vi "Get Screen BD Object Bounds.vi"(9 "Object Reference":refnum<vi>, 10 "BD Window Bounds":T1, 11 "BD Origin":T2) -> (1 "Object Visible?":bool, 2 "Screen Object Bounds":T1, 3 "Screen BD Bounds":T1)   [LabVIEW 2019, in "Window.lvlib"]
doc: "Converts the given block diagram coordinates into screen coordinates. Also converts the given object's size and position from block diagram coordinates to screen coordinates. The object is also checked for visibility on the block diagram window."
uses:
  <vilib>/Utility/miscctls.llb/LVPointTypeDef.ctl
  <vilib>/Utility/miscctls.llb/LVRectTypeDef.ctl
  Window.lvlib
  _2D/2D.lvlib
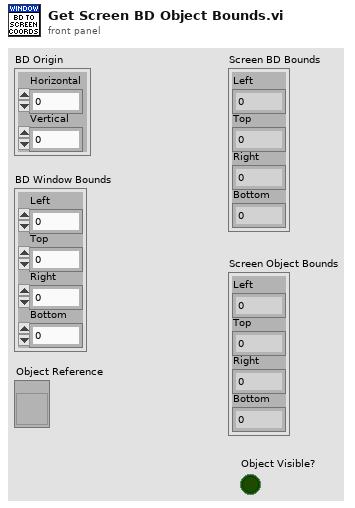
[diagram p1: front panel]
types:
  T1 = typedef "LVRectTypeDef.ctl" = cluster{"Left":i16, "Top":i16, "Right":i16, "Bottom":i16}
  T2 = typedef "LVPointTypeDef.ctl" = cluster{"Horizontal":i16, "Vertical":i16}
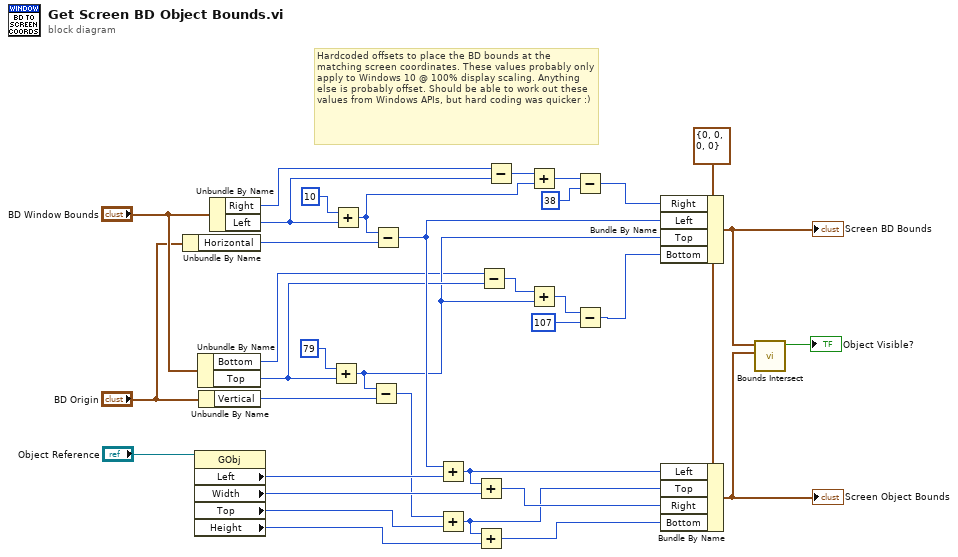
[diagram p0: block diagram]
diagram:
  w26 = T1 {"Left"=0, "Top"=0, "Right"=0, "Bottom"=0} ("Screen BD Bounds")
  # "Hardcoded offsets to place the BD bounds at the matching screen coordinates. These values probably only apply to Windows 10 @ 100% display scaling. Anything else is probably offset. Should be able to work out these values from Windows APIs, but hard coding was quicker :)"
  n1 = Unbundle By Name("BD Origin") -> ("Horizontal"=w29:i16)
  n2 = property class="GObj"(reference="Object Reference") -> ("Left"=w33:i32, "Width"=w32:u32, "Top"=w31:i32, "Height"=w30:u32)  [unwired: 1 in, 2 out]
  n3 = Unbundle By Name("BD Window Bounds") -> ("Bottom"=w5:i16, "Top"=w15:i16)
  n4 = Unbundle By Name("BD Origin") -> ("Vertical"=w27:i16)
  n5 = Unbundle By Name("BD Window Bounds") -> ("Right"=w6:i16, "Left"=w19:i16)
  n6 = Add(x=i16 79 ("y"), y=w15) -> (x+y=w13:i16)
  n7 = Add(x=i16 10, y=w19) -> (x+y=w7:i16)
  n8 = Subtract(x=w13, y=w27) -> (x-y=w20:i16)
  n9 = Subtract(x=w7, y=w29) -> (x-y=w21:i16)
  n10 = Add(x=w21, y=w33) -> (x+y=w25:i32)
  n11 = Add(x=w20, y=w31) -> (x+y=w23:i32)
  n12 = Add(x=w25, y=w32) -> (x+y=w24:u32)
  n13 = Add(x=w23, y=w30) -> (x+y=w22:u32)
  n14 = Subtract(x=w5, y=w15) -> (x-y=w14:i16)
  n15 = Subtract(x=w6, y=w19) -> (x-y=w18:i16)
  n16 = Add(x=w18, y=w7) -> (x+y=w17:i16)
  n17 = Add(x=w14, y=w13) -> (x+y=w12:i16)
  n18 = Subtract(x=w17, y=i16 38) -> (x-y=w8:i16)
  n19 = Subtract(x=w12, y=i16 107) -> (x-y=w4:i16)
  n20 = Bundle By Name(cluster=w26, "Right"=w8, "Left"=w21, "Top"=w13, "Bottom"=w4) -> (w3:T1)
  "Screen BD Bounds" <- w3
  n21 = Bundle By Name(cluster=w26, "Left"=w25, "Top"=w23, "Right"=w24, "Bottom"=w22) -> (w2:T1)
  "Screen Object Bounds" <- w2
  n22 = call "Bounds Intersect.vi"("Bounds 2"=w2, "Bounds 1"=w3) -> ("Intersect?"=→"Object Visible?":bool)  [unwired: 9 in]
